vi "sedSpectrometer_monitorCommand_captureSpectImage.vi"(8 "error in (no error)":errorcluster, 11 "command_captureSpectImage_Ctl":T1={"integrationTime"=0.0, "imageType"="                                                                                                                                                                                                                                                                ", "lamp"=""}) -> (0 "error out":errorcluster, 2 "function return":i32, 3 "command_captureSpectImage_Ctl out":T1={"integrationTime"=0.0, "imageType"="                                                                                                                                                                                                                                                                ", "lamp"=""})   [LabVIEW 2016, in "SALLV_sedSpectrometer.lvlib"]
doc: "int sedSpectrometer_shm_monitorCommand_captureSpectImageLV(sedSpectrometer_command_captureSpectImageLV *command_captureSpectImage_Ctl );"
uses:
  SALLV_sedSpectrometer.lvlib
  DataTypes/command_captureSpectImage.ctl
  SALLV_sedSpectrometer.so
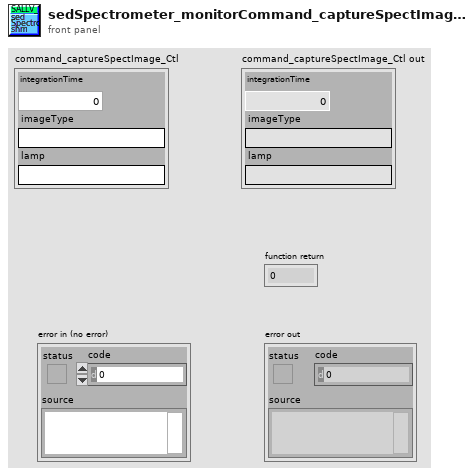
[diagram p1: front panel]
types:
  T1 = typedef "SALLV_sedSpectrometer.lvlib/command_captureSpectImage.ctl" = cluster{"integrationTime":sgl, "imageType":string, "lamp":string}
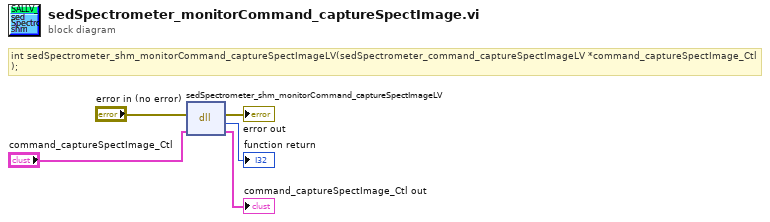
[diagram p0: block diagram]
diagram:
  # "int sedSpectrometer_shm_monitorCommand_captureSpectImageLV(sedSpectrometer_command_captureSpectImageLV *command_captureSpectImage_Ctl );"
  n1 = dll-call lib="home/harini/TCS/ts_sallv_sedSpectrometer/SALLV_sedSpectrometer.*" fn="sedSpectrometer_shm_monitorCommand_captureSpectImageLV"(error in="error in (no error)", "command_captureSpectImage_Ctl"="command_captureSpectImage_Ctl") -> (error out=→"error out":errorcluster, →"function return":i32, "command_captureSpectImage_Ctl"=→"command_captureSpectImage_Ctl out":T1)  [unwired: 2 in, 1 out]
